vi "main.vi"() -> ()   [LabVIEW 2010]
uses:
  <vilib>/Platform/TimedLoop/XDataNode/XDataNode.xnode
  <vilib>/Platform/TimedLoop/XDataNode/timing_clust.ctl
  <vilib>/Platform/TimedLoop/XDataNode/nitl_modes.ctl
  <vilib>/Platform/TimedLoop/XDataNode/wakeup.ctl
  <vilib>/rvi/DataTransferAndStorage/Container/XNode/niFpgaContainer.xnode
  <vilib>/eio/EIONode/EIONode.xnode
  <vilib>/rvi/eio/nirviEIOImplementation/nirviEIOImplementation.xnode
  <vilib>/rvi/eio/common/nirviEmuClasses.ctl
  <vilib>/rvi/DataTransferAndStorage/Container/Common/niFpgaContainerMethod.ctl
  <vilib>/rvi/DataTransferAndStorage/Container/Common/niFpgaTransferTypeControl.ctl
  <vilib>/rvi/FIFO/Fifo_Resource/nirvififoEmulationSetSize.vi
  <vilib>/rvi/DataTransferAndStorage/Container/Common/niFpgaContainerGetUniqueNameForEmu.vi
  <vilib>/rvi/eio/common/nirviEmuTemplateMethod_noerrors.vi
  <vilib>/rvi/Memory/Memory_Emulation/nirvimemoryEmulationManagerCache_GetValue.vi
  <vilib>/rvi/Memory/Memory_Emulation/nirvimemoryEmulationManagerCache_InsertValue.vi
  <vilib>/Utility/error.llb/Clear Errors.vi
  <vilib>/rvi/Memory/Memory_Emulation/nirvimemoryEmulationManagerCache_SetValue.vi
  <vilib>/rvi/interface/RandomDataEmulation/nirviRandomDataFPGAFIFO.vi
  <vilib>/rvi/interface/RandomDataEmulation/niFpgaRandomDataHandleErrors.vi
  <vilib>/Platform/TimedLoop/XDataNode/XDNodeRunTimeDep.lvlib
panel:
  out "last address sent":u16
  in  "transmit address":bool
  out "last address zeroed":u16
  out "fifo to host overflow":bool
  in  "slow mod":bool
  in  "integration counts":u16=3
  in  "stim delay":u16
  out "elements queued in fifo":u32
  out "Timed Out?":bool
  out "photons sent loop2loop":u32
  out "ch0 photons loop2loop":u32
  out "ch0 photons sent":u32
  out "total photons ch0":u32
  out "counter":u16
  out "address":u16
  in  "stop":bool
  out "sweeps counted":u32
  in  "stim enable":bool
  in  "stim counts":u16
  in  "count photons":bool
  in  "cycle width":u16
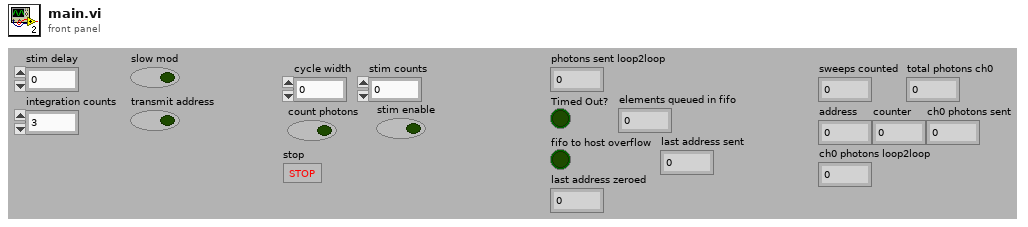
[diagram p1: front panel]
types:
  T1 = typedef "XDNodeRunTimeDep.lvlib/timing_clust.ctl" = cluster{"Expected End [f-1]":u64, "Actual End [f-1]":u64, "Finished Late? [f-1]":bool, "Expected End [i-1]":u64, "Actual End [i-1]":u64, "Finished Late? [i-1]":bool, "Expected Start [i]":u64, "Actual Start [i]":u64, "Expected Start [f]":u64, "Actual Start [f]":u64, "Source Name":string, "Structure Name":string, "Period":i64, "Deadline":i64, "Offset":i64, "Start":i64, "Priority":i32, "Timeout":i32, "Mode":T2, "Wakeup Reason":T3, "Error":errorcluster, "Source Type":string, "Secondary Source Type":string, "Global End Time":u64, "Global Start Time":u64, "Frame Duration":u64, "Iteration Duration":u64, "Assigned CPU":i32, "I/O Scan Engine Mode":u32}
  T2 = typedef "XDNodeRunTimeDep.lvlib/nitl_modes.ctl" = enum32{"No Change", "Process missed periods, maintain original phase", "Discard missed periods, maintain original phase", "Process missed periods, ignore original phase", "Discard missed periods, ignore original phase"}
  T3 = typedef "XDNodeRunTimeDep.lvlib/wakeup.ctl" = enum32{"Normal", "Aborted", "Asynchronous wakeup", "Timing source error", "Timed loop error", "Timeout"}
  T4 = typedef "nirviEmuClasses.ctl" = enum16{"IO Read", "IO Write", "Method", "Property Read", "Property Write"}
  T5 = typedef "niFpgaContainerMethod.ctl" = enum16{"<none>", "write", "read", "clear", "getNumberOfElementsToWrite", "getNumberOfElementsToRead", "enable", "disable", "flushAndDisable", "getStreamState", "readA", "readB", "dramWrite", "dramWriteWithByteEnables", "dramRequestData", "dramRetrieveData"}
  T6 = typedef "niFpgaTransferTypeControl.ctl" = enum16{"Target-Scoped", "Host to Target - DMA", "Target to Host - DMA", "Peer to Peer Reader", "Peer to Peer Writer", "Bidirectional"}
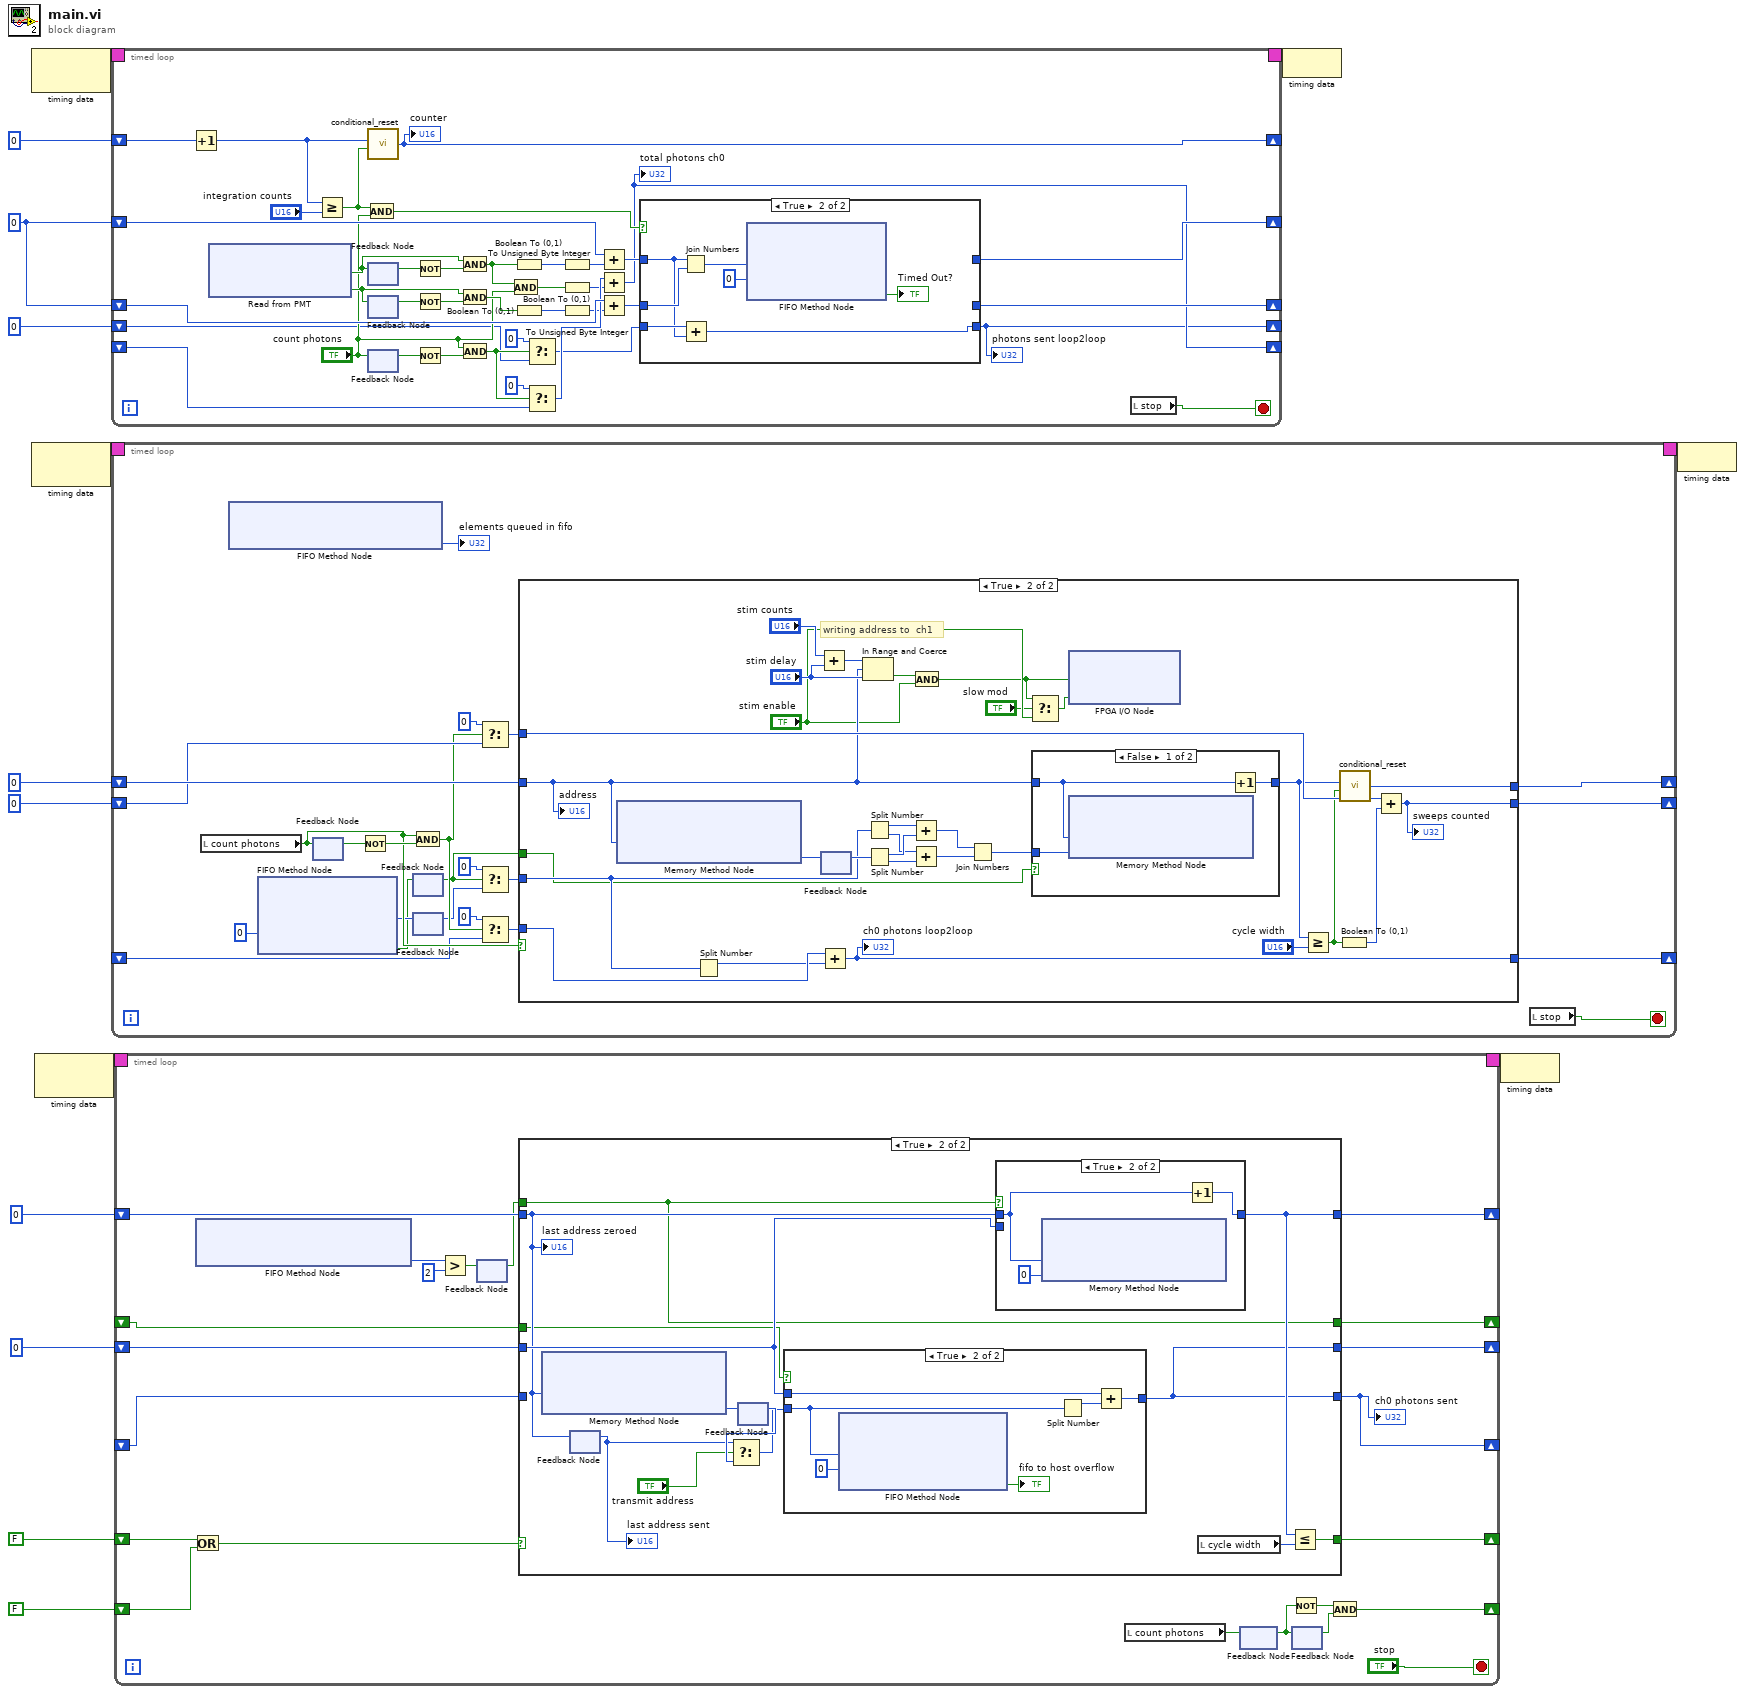
[diagram p0: block diagram]
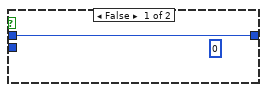
[diagram p4: hidden frame]
diagram:
  w7 = u8 0
  n1 = node-c288() -> (w15:T1)  [unwired: 1 in]
  n2 = node-c288() -> (w12:T1)  [unwired: 1 in]
  n3 = node-c288() -> (w2:T1)  [unwired: 1 in]
  n4 = timed-loop {
    timing: w15 -> [_]
    timing-out: [_] -> w14
    shift-right: [w45] -> _
    shift-left: u8 0 -> [w48]
    shift-right: [w36] -> _
    shift-left: w7 -> [w40]
    shift-right: [w37] -> _
    shift-left: w7 -> [w42]
    shift-right: [w28] -> _
    shift-left: _ -> [w27]
    shift-right: [w19] -> _
    shift-left: i16 0 -> [w18]
    stop <- w34 stop-if-true
    n5 = Increment(x=w48) -> (x+1=w47:u16)
    n6 = xnode "Read from PMT"() -> ("Connector1/DIO23"=w53:bool, "Connector1/DIO1"=w49:bool)  [unwired: 2 in, 2 out]
    n7 = Greater Or Equal?(x=w47, y="integration counts") -> (x >= y?=w44:bool)
    n8 = And(x=w44, y="count photons") -> (x .and. y?=w35:bool)
    n9 = call "conditional_reset.vi"("reset?"=w44, "number in"=w47) -> ("number out"=w45:u16)  [unwired: 4 in]
    "counter" <- w45
    n10 = feedback-in #1(w53) -> ()
    n11 = feedback #1() -> (w52:bool)  [unwired: 1 in]
    n12 = feedback #2() -> (w50:bool)  [unwired: 1 in]
    n13 = feedback-in #2(w49) -> ()
    n14 = feedback #3() -> (w33:bool)  [unwired: 1 in]
    n15 = feedback-in #3("count photons") -> ()
    n16 = Not(x=w52) -> (.not. x?=w54:bool)
    n17 = Not(x=w50) -> (.not. x?=w51:bool)
    n18 = Not(x=w33) -> (.not. x?=w32:bool)
    n19 = And(x=w53, y=w54) -> (x .and. y?=w26:bool)
    n20 = And(x=w49, y=w51) -> (x .and. y?=w43:bool)
    n21 = And(x="count photons", y=w32) -> (x .and. y?=w22:bool)
    n22 = And(x=w26, y="count photons") -> (x .and. y?=w24:bool)
    n23 = Boolean To (0,1)(Boolean=w26) -> (0, 1=w29:i16)
    n24 = Boolean To (0,1)(Boolean=w43) -> (0, 1=w41:i16)
    n25 = Select(t=u32 0, s=w22, f=w18) -> (s? t:f=w20:u32)
    n26 = Select(t=u32 0, s=w22, f=w27) -> (s? t:f=w30:u32)
    n27 = To Unsigned Byte Integer(number=w29) -> (unsigned 8bit integer=w17:u8)
    n28 = Boolean To (0,1)(Boolean=w24) -> (0, 1=w23:i16)
    n29 = To Unsigned Byte Integer(number=w41) -> (unsigned 8bit integer=w16:u8)
    n30 = Add(x=w42, y=w17) -> (x+y=w38:u8)
    n31 = Add(x=w30, y=w23) -> (x+y=w28:u32)
    "total photons ch0" <- w28
    n32 = Add(x=w40, y=w16) -> (x+y=w39:u8)
    n33 = case shown="True" w35 {
      tunnel: w39 -> [w56 w63]
      tunnel: w38 -> [w57 w60]
      tunnel: [w57 _] -> w37
      tunnel: [w56 _] -> w36
      tunnel: w20 -> [w55 w61]
      tunnel: [w55 w59] -> w19
      frame False {
      }
      frame True {
        n34 = Join Numbers(hi=w60, lo=w63) -> ((hi.lo)=w62:u16)
        n35 = Add(x=w61, y=w60) -> (x+y=w59:u32)
        n36 = xnode ("FIFO Method Node")("Element"=w62, "Timeout"=0) -> ("Timed Out?"=→"Timed Out?":bool)  [unwired: 1 in, 1 out]
      }
    }
    "photons sent loop2loop" <- w19
    n37 = local read "stop"() -> (w34:bool)
  }
  n38 = timed-loop {
    timing: w12 -> [_]
    timing-out: [_] -> w11
    shift-right: [w178] -> _
    shift-left: u16 0 -> [w175]
    shift-right: [w177] -> _
    shift-left: u32 0 ("number out") -> [w170]
    shift-right: [w162] -> _
    shift-left: _ -> [w161]
    stop <- w176 stop-if-true
    n39 = local read "count photons"() -> (w172:bool)
    n40 = xnode ("FIFO Method Node")() -> ("Number of Elements to Read"=→"elements queued in fifo":u32)  [unwired: 1 in, 1 out]
    n41 = xnode ("FIFO Method Node")("Timeout"=0) -> ("Element"=w168:u16, "Timed Out?"=w166:bool)  [unwired: 1 in, 1 out]
    n42 = feedback #4() -> (w174:bool)  [unwired: 1 in]
    n43 = feedback-in #4(w172) -> ()
    n44 = Not(x=w174) -> (.not. x?=w173:bool)
    n45 = And(x=w172, y=w173) -> (x .and. y?=w165:bool)
    n46 = feedback-in #5(w166) -> ()
    n47 = feedback #5() -> (w156:bool)  [unwired: 1 in]
    n48 = feedback #6() -> (w158:u16)  [unwired: 1 in]
    n49 = feedback-in #6(w168) -> ()
    n50 = Select(t=u32 0, s=w165, f=w170) -> (s? t:f=w171:u32)
    n51 = Select(t=u16 0 ("f"), s=w156, f=w158) -> (s? t:f=w159:u16)
    n52 = Select(t=u32 0, s=w165, f=w161) -> (s? t:f=w163:u32)
    n53 = case shown="True" w172 {
      tunnel: [_ w283] -> w178
      tunnel: w175 -> [_ w282]
      tunnel: [w274 w297] -> w177
      tunnel: w171 -> [w274 w294]
      tunnel: w159 -> [_ w292]
      tunnel: w156 -> [_ w289]
      tunnel: w163 -> [w273 w293]
      tunnel: [w273 w290] -> w162
      frame False {
      }
      frame True {
        # "writing address to  ch1"
        n54 = xnode ("Memory Method Node")("Address"=w282) -> ("Data"=w296:u64)  [unwired: 1 in, 1 out]
        n55 = Split Number(x=w292) -> (hi(x)=w291:u8)  [unwired: 1 out]
        n56 = Add(x="stim counts", y="stim delay") -> (x+y=w287:u16)
        n57 = Add(x=w293, y=w291) -> (x+y=w290:u32)
        "ch0 photons loop2loop" <- w290
        n58 = feedback #7() -> (w295:u64)  [unwired: 1 in]
        n59 = feedback-in #7(w296) -> ()
        n60 = In Range and Coerce(upper limit=w287, x=w282, lower limit="stim delay") -> (In Range?=w285:bool)  [unwired: 1 out]
        n61 = Split Number(x=w292) -> (hi(x)=w304:u8, lo(x)=w302:u8)
        n62 = Split Number(x=w295) -> (hi(x)=w303:u32, lo(x)=w301:u32)
        n63 = Add(x=w304, y=w303) -> (x+y=w300:u32)
        n64 = Add(x=w302, y=w301) -> (x+y=w284:u32)
        n65 = And(x=w285, y="stim enable") -> (x .and. y?=w279:bool)
        n66 = Join Numbers(hi=w300, lo=w284) -> ((hi.lo)=w299:u64)
        n67 = Select(t=w279, s="slow mod", f="stim enable") -> (s? t:f=w277:bool)
        n68 = case shown="False" w289 {
          tunnel: w282 -> [w454 w581]
          tunnel: w299 -> [w455 _]
          tunnel: [w453 w581] -> w275
          frame False {
            n69 = xnode ("Memory Method Node")("Address"=w454, "Data"=w455) -> ()  [unwired: 1 in, 1 out]
            n70 = Increment(x=w454) -> (x+1=w453:u16)
          }
          frame True {
          }
        }
        n71 = xnode "FPGA I/O Node"("stim window"=w279, "stim enable"=w277) -> ()  [unwired: 2 in, 2 out]
        n72 = Greater Or Equal?(x=w275, y="cycle width") -> (x >= y?=w281:bool)
        n73 = Boolean To (0,1)(Boolean=w281) -> (0, 1=w298:i16)
        n74 = call "conditional_reset.vi"("reset?"=w281, "number in"=w275) -> ("number out"=w283:u16)  [unwired: 4 in]
        n75 = Add(x=w294, y=w298) -> (x+y=w297:u32)
        "sweeps counted" <- w297
        "address" <- w282
      }
    }
    n76 = local read "stop"() -> (w176:bool)
  }
  n77 = timed-loop {
    shift-right: [w605] -> _
    shift-left: u16 0 -> [w604]
    shift-right: [w603] -> _
    shift-left: u32 0 -> [w602]
    shift-right: [w597] -> _
    shift-left: FALSE -> [w595]
    shift-right: [w598] -> _
    shift-left: FALSE -> [w594]
    timing: w2 -> [_]
    timing-out: [_] -> w1
    shift-right: [w587] -> _
    shift-left: _ -> [w586]
    shift-right: [w585] -> _
    shift-left: _ -> [w584]
    stop <- "stop" stop-if-true
    n78 = Or(x=w595, y=w594) -> (x .or. y?=w593:bool)
    n79 = xnode ("FIFO Method Node")() -> ("Number of Elements to Write"=w590:u32)  [unwired: 1 in, 1 out]
    n80 = Greater?(x=w590, y=u32 2) -> (0:w589:bool)
    n81 = feedback #8() -> (w588:bool)  [unwired: 1 in]
    n82 = feedback-in #8(w589) -> ()
    n83 = case shown="True" w593 {
      tunnel: [_ w636] -> w603
      tunnel: [_ w644] -> w605
      tunnel: w604 -> [_ w640]
      tunnel: w602 -> [_ w642]
      tunnel: [_ w643] -> w597
      tunnel: w588 -> [_ w635]
      tunnel: [w633 w636] -> w587
      tunnel: w586 -> [w633 _]
      tunnel: [_ w635] -> w585
      tunnel: w584 -> [_ w634]
      frame False {
      }
      frame True {
        n84 = xnode ("Memory Method Node")("Address"=w640) -> ("Data"=w646:u64)  [unwired: 1 in, 1 out]
        n85 = feedback #9() -> (w639:u16)  [unwired: 1 in]
        "last address sent" <- w639
        n86 = feedback-in #9(w640) -> ()
        n87 = feedback #10() -> (w641:u64)  [unwired: 1 in]
        n88 = Select(t=w639, s="transmit address", f=w641) -> (s? t:f=w638:u64)
        n89 = feedback-in #10(w646) -> ()
        n90 = case shown="True" w634 {
          tunnel: [w647 w650] -> w636
          tunnel: w642 -> [w647 w649]
          tunnel: w638 -> [_ w648]
          frame False {
          }
          frame True {
            n91 = xnode ("FIFO Method Node")("Element"=w648, "Timeout"=0) -> ("Timed Out?"=→"fifo to host overflow":bool)  [unwired: 1 in, 1 out]
            n92 = Split Number(x=w648) -> (hi(x)=w651:u32)  [unwired: 1 out]
            n93 = Add(x=w649, y=w651) -> (x+y=w650:u32)
          }
        }
        n94 = case shown="True" w635 {
          tunnel: w640 -> [w682 w684]
          tunnel: w642 -> [_ _]
          tunnel: [w682 w683] -> w644
          frame False {
            (unwired) u32 0
          }
          frame True {
            n95 = xnode ("Memory Method Node")("Address"=w684, "Data"=u64 0) -> ()  [unwired: 1 in, 1 out]
            n96 = Increment(x=w684) -> (x+1=w683:u16)
          }
        }
        n97 = local read "cycle width"() -> (w645:u16)
        n98 = Less Or Equal?(x=w644, y=w645) -> (x <= y?=w643:bool)
        "last address zeroed" <- w640
      }
    }
    "ch0 photons sent" <- w587
    n99 = local read "count photons"() -> (w599:bool)
    n100 = feedback #11() -> (w596:bool)  [unwired: 1 in]
    n101 = feedback-in #11(w599) -> ()
    n102 = Not(x=w596) -> (.not. x?=w601:bool)
    n103 = feedback #12() -> (w600:bool)  [unwired: 1 in]
    n104 = feedback-in #12(w596) -> ()
    n105 = And(x=w601, y=w600) -> (x .and. y?=w598:bool)
  }
  n106 = node-c288(w14) -> ()
  n107 = node-c288(w1) -> ()
  n108 = node-c288(w11) -> ()
